vi "Close.vi"(0 "Power Detector in":refnum<class "Power Detector.lvclass">, 11 "error in":errorcluster) -> (4 "Power Detector out":refnum<class "Power Detector.lvclass">, 15 "error out":errorcluster)   [LabVIEW 2023, in "NI CAL-5501 Power Detector.lvlib" / "Power Detector.lvclass"]
uses:
  Power Detector.lvclass
  Power Detector.lvclass/Power Detector.ctl
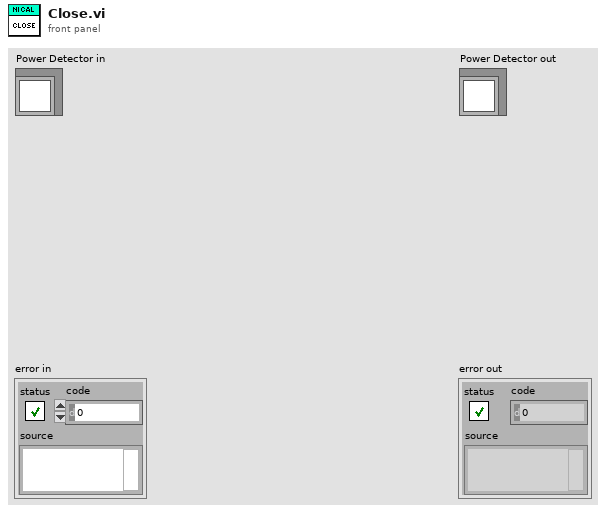
[diagram p1: front panel]
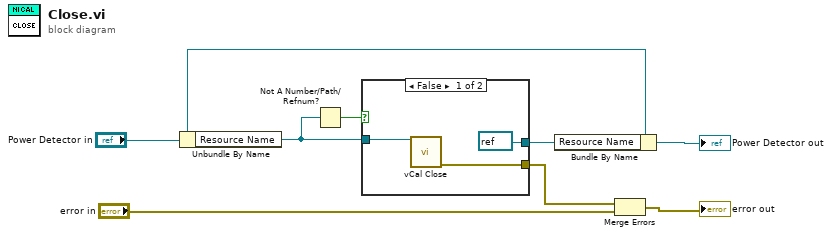
[diagram p0: block diagram]
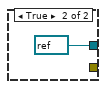
[diagram p2: hidden frame]
diagram:
  n1 = Unbundle By Name("Power Detector in") -> ("Resource Name"=w4:refnum<k15>)
  n2 = Not A Number/Path/Refnum?(number/path/refnum=w4) -> (NaN/Path/Refnum?=w5:bool)
  n3 = case shown="False" w5 {
    tunnel: w4 -> [w11 _]
    tunnel: [w10 _] -> w2
    tunnel: [refnum<k15> refnum ("Resource Name") refnum<k15> refnum ("Resource Name")] -> w3
    frame False {
      n4 = call <instrlib>:"vCal Close.vi"("instrument handle"=w11) -> ("error out"=w10:errorcluster)  [unwired: 14 in]
    }
    frame True {
    }
  }
  n5 = Bundle By Name(cluster="Power Detector in", "Resource Name"=w3) -> (→"Power Detector out":refnum<class "Power Detector.lvclass">)
  n6 = Merge Errors(w2, "error in") -> (→"error out":errorcluster)
